vi "Accelerator Read RF Bin quick record 2020 all exec without indicator and warmup.vi"(9 "Sessions Parameters":T2 {"graph_optimization_level" items=["ORT_DISABLE_ALL"=0, "ORT_ENABLE_ALL"=1, "ORT_ENABLE_BASIC"=2, "ORT_ENABLE_EXTENDED"=99]}, 10 "Execution Device":T1=enum."TensorRT", 11 "file path":path=path "C:/Users/COCO/Desktop/TEMP.BIN") -> (3 "exec time":dbl)   [LabVIEW 2020]
uses:
  Source/_Controls/acc_execution_provider_enum.ctl
  Source/Layer/Node/_Controls/acc_onnx_dtype_enum.ctl
  Source/Model/Controls/acc_input_parameters.ctl
  Source/ONNX/_Controls/acc_CUDA_ep_params_simplified.ctl
  Source/ONNX/_Controls/acc_tensorRT_ep_params_simplified.ctl
  Source/Model/_Methods/add_to_graph/Initializer/acc_float_scalar_initializer.vi
  Source/Model/_Methods/add_to_graph/Numeric/acc_div_adaptive.vi
  Source/Model/_Methods/add_to_graph/Complex/Transforms/acc_FFT_optimized.vi
  Source/Model/_Methods/add_to_graph/Initializer/acc_complexfloat_scalar_initializer.vi
  Source/Model/_Methods/add_to_graph/Numeric/acc_mul_adaptive.vi
  Source/Model/_Methods/add_to_graph/Numeric/acc_add_adaptive.vi
  Source/SubVIs/acc_open_netron_from_labview_model.vi
  Source/Model/_Methods/acc_create_onnx_model_then_init_cuda_inference_session.vi
  Source/Model/_Methods/acc_create_onnx_model_then_init_inference_session.vi
  Source/Model/_Methods/acc_create_onnx_model_then_init_tensorRT_inference_session.vi
  Source/ONNX/Inference/_Methods/Simplified/acc_embedded_run_preallocated_mono_input_and_outputs_gpu_by_idx.vi
  Source/ONNX/Inference/_Methods/Exec_GPU/acc_embedded_copy_ptr_data_to_labview_data.vi
  Source/ONNX/Inference/_Methods/Simplified/acc_embedded_run_mono_output_1d_float.vi
  Source/ONNX/Inference/acc_Inference.lvclass
  Source/Model/acc_Model.lvclass
panel:
  out "error out":errorcluster
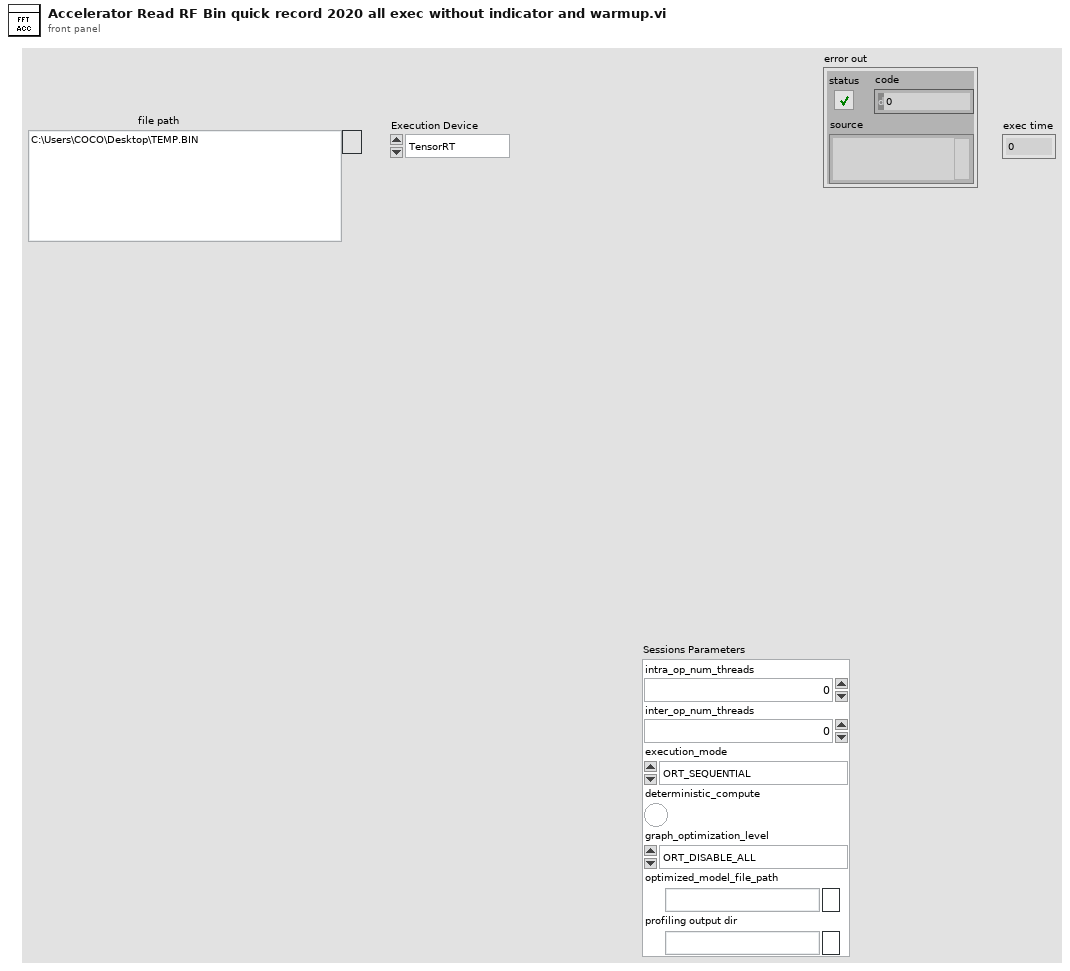
[diagram p1: front panel]
types:
  T1 = typedef "acc_execution_provider_enum.ctl" = enum16{"CPU", "CUDA", "TensorRT"}
  T2 = cluster{"intra_op_num_threads":i32, "inter_op_num_threads":i32, "execution_mode":enum16{"ORT_SEQUENTIAL", "ORT_PARALLEL"}, "deterministic_compute":bool, "graph_optimization_level":u16, "optimized_model_file_path":path, "profiling output dir":path}
  T3 = typedef "acc_input_parameters.ctl" = cluster{"Rank":enum16{"Scalar", "1D", "2D", "3D", "4D", "5D", "6D"}, "dtype":T4, "complex?":bool, "expert?":bool}
  T4 = typedef "acc_onnx_dtype_enum.ctl" = enum16{"UNDEFINED", "FLOAT", "UINT8", "INT8", "UINT16", "INT16", "INT32", "INT64", "STRING", "BOOL", "FLOAT16", "DOUBLE", "UINT32", "UINT64", "COMPLEX64", "COMPLEX128", "BFLOAT16", "FLOAT8E4M3FN", "FLOAT8E4M3FNUZ", "FLOAT8E5M2", "FLOAT8E5M2FNUZ", "UINT4", "INT4"}
  T5 = cluster{"inputs_ptr":u64, "inputs_shapes":i64[], "inputs_ranks":i64, "inputs_types":T4}
  T6 = cluster{"outputs_ptr":u64, "outputs_shapes":i64[], "outputs_ranks":i64, "outputs_types":T4}
  T7 = enum16{"open", "replace", "create", "open or create", "replace or create", "replace or create with confirmation"}
  T8 = typedef "acc_CUDA_ep_params_simplified.ctl" = cluster{"Device & Stream":cluster{"Device Index":i32, "Use Custom Compute Stream?":bool, "Custom Compute Stream (Pointer)":u64, "Copy Using Default Stream?":bool}, "Memory Management":cluster{"GPU Memory Limit (Bytes)":u64, "Arena Extension Strategy":enum16{"kNextPowerOfTwo", "kSameAsRequested"}, "Default Memory Arena Config":u64}, "CuDNN & Kernel Optimization":cluster{"cuDNN Convolution Algorithm Search":enum16{"OrtCudnnConvAlgoSearchExhaustive", "OrtCudnnConvAlgoSearchHeuristic", "OrtCudnnConvAlgoSearchDefault"}, "Use Max Workspace for cuDNN?":bool, "Pad Conv1D Inputs to NC1D?":bool, "Fuse Convolution + Bias?":bool, "Scaled Dot-Product Attention Kernel Option":bool, "Enable Strict SkipLayerNorm Mode?":bool}, "Execution & Precision Controls":cluster{"Enable CUDA Graph Execution?":bool, "Use EP-Level Unified Stream?":bool, "Prefer NHWC Tensor Layout?":bool, "Use TensorFloat-32 (TF32)?":bool}, "Tunable Operator System":cluster{"Enable Tunable Operators?":bool, "Enable Tuning Mode for Tunable Operators?":bool, "Max Tuning Duration (ms)":i32}}
  T9 = typedef "acc_tensorRT_ep_params_simplified.ctl" = cluster{"Device And Stream":cluster{"Device Index":i32, "Use Custom Compute Stream?":bool, "Custom Compute Stream (Pointer)":u64}, "Parser & Subgraph Options":cluster{"Max Partition Attemps":i32, "Minimum Subgraph Size":i32}, "Memory & Workspace Management":cluster{"Max Workspace Memory (Bytes)":u64, "Share Memory Between Subgraphs":bool, "Auxiliary Stream Count":i32}, "Precision & Numeric Modes":cluster{"Enable FP16":bool, "Enable BF16":bool, "Enable INT8":bool, "INT8 Calibration Table Name":path, "Use Native INT8 Calibration?":bool}, "Engine Build, Cache & Paths":cluster{"Enable Engine Caching?":bool, "Engine Cache Directory":path, "Enable Engine Decryption?":bool, "Decryption Library Path":path, "Build Engines Sequentially?":bool, "Enable Timing Cache?":bool, "Timing Cache Directory":path, "Force Timing Cache Use?":bool, "Enable Detailed Logs?":bool, "Use Build Heuristics?":bool, "Enable Weight Sparsity?":bool, "Engine Optimization Level (0–5)":i32}, "Paths & Plugins":cluster{"Extra Plugin Libraries":path[], "Tactic Source Rules":string, "Enabled Preview Features":enum16{"None", "ALIASED_PLUGIN_IO_10_03"}}, "Profile Shapes":cluster{"Minimum Input Shapes":string, "Maximum Input Shapes":string, "Optimal Input Shapes":string}, "Advanced & DLA / CUDA Graph":cluster{"Enable DLA Acceleration?":bool, "DLA Core Index":i32, "Dump TensorRT Subgraphs?":bool, "Force LayerNorm in FP32?":bool, "Enable CUDA Graph Execution?":bool}}
  T10 = enum16{"big-endian, network order", "native, host order", "little-endian"}
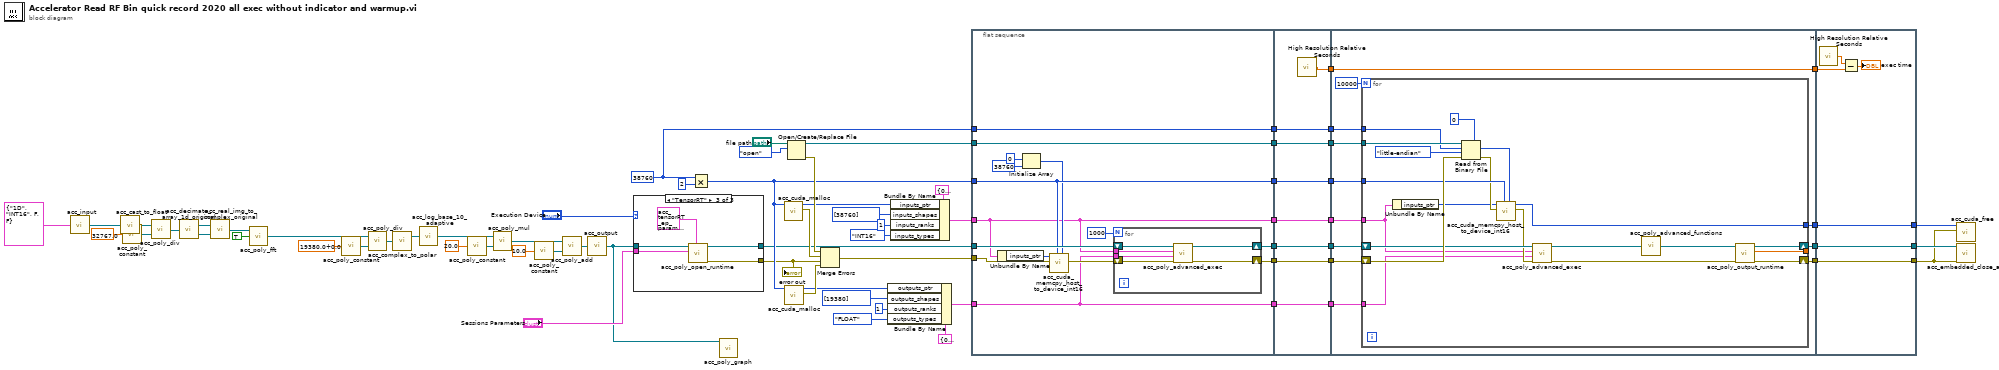
[diagram p0: block diagram]
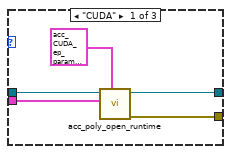
[diagram p2: hidden frame]
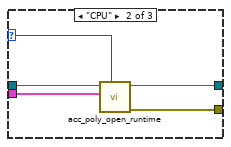
[diagram p3: hidden frame]
diagram:
  w64 = 38760 ("count (1)")
  n1 = call "acc_input.vi"("Parameters"=T3 {"Rank"=enum."1D", "dtype"=enum."INT16", "complex?"=FALSE, "expert?"=FALSE}) -> ("ONNXModel out"=w34:refnum<class "acc_Model.lvclass">)  [unwired: 8 in]
  n2 = call "acc_cast_to_float.vi"("x"=w34) -> ("sgl(x)"=w18:refnum<class "acc_Model.lvclass">)
  n3 = call-poly "acc_poly_constant.vi"("scalar"=sgl 32767.0 ("Numeric")) -> ("Float Scalar"=w16:refnum<class "acc_Model.lvclass">)  [unwired: 3 in]
  n4 = call-poly "acc_poly_div.vi"("y"=w16, "x"=w18) -> ("x/y"=w19:refnum<class "acc_Model.lvclass">)
  n5 = call "acc_decimate_array_1d_original.vi"("array"=w19) -> ("elements 0, n, 2n"=w21:refnum<class "acc_Model.lvclass">, "elements 1, n+1, 2n+1"=w20:refnum<class "acc_Model.lvclass">)
  n6 = call "acc_real_img_to_complex_original.vi"("y"=w20, "x"=w21) -> ("x + iy"=w33:refnum<class "acc_Model.lvclass">)
  n7 = call-poly "acc_poly_fft.vi"("shift?"=TRUE, "X"=w33) -> ("FFT {X}"=w32:refnum<class "acc_Model.lvclass">)  [unwired: 1 in]
  n8 = call-poly "acc_poly_constant.vi"("scalar"=csg 19380.0+0.0i ("Numeric")) -> ("Complex Float Scalar"=w13:refnum<class "acc_Model.lvclass">)  [unwired: 3 in]
  n9 = call-poly "acc_poly_div.vi"("y"=w13, "x"=w32) -> ("x/y"=w26:refnum<class "acc_Model.lvclass">)
  n10 = call "acc_complex_to_polar.vi"("r * e^(i*theta)"=w26) -> ("r"=w22:refnum<class "acc_Model.lvclass">)  [unwired: 1 out]
  n11 = call "acc_log_base_10_adaptive.vi"("x"=w22) -> ("log(x)"=w31:refnum<class "acc_Model.lvclass">)
  n12 = call-poly "acc_poly_constant.vi"("scalar"=sgl 20.0 ("Numeric")) -> ("Float Scalar"=w24:refnum<class "acc_Model.lvclass">)  [unwired: 3 in]
  n13 = call-poly "acc_poly_mul.vi"("y"=w24, "x"=w31) -> ("x*y"=w29:refnum<class "acc_Model.lvclass">)
  n14 = call-poly "acc_poly_constant.vi"("scalar"=sgl 10.0 ("Numeric")) -> ("Float Scalar"=w23:refnum<class "acc_Model.lvclass">)  [unwired: 3 in]
  n15 = call-poly "acc_poly_add.vi"("y"=w23, "x"=w29) -> ("x+y"=w25:refnum<class "acc_Model.lvclass">)
  n16 = call "acc_output.vi"("ONNXModel in"=w25) -> ("ONNXModel out"=w1:refnum<class "acc_Model.lvclass">)  [unwired: 8 in]
  n17 = case shown="\"TensorRT\"" "Execution Device" {
    selector: "Execution Device" -> [_ w77 _]
    tunnel: [w76 w81 w86] -> w5
    tunnel: [w75 w80 w85] -> w4
    tunnel: "Sessions Parameters" -> [w74 w79 w84]
    tunnel: w1 -> [w73 w78 w83]
    frame "CUDA" {
      n18 = call-poly "acc_poly_open_runtime.vi"("CUDA Parameters"=T8 {"Device & Stream"={"Device Index"=0, "Use Custom Compute Stream?"=FALSE, "Custom Compute Stream (Pointer)"=0, "Copy Using Default Stream?"=TRUE}, "Memory Management"={"GPU Memory Limit (Bytes)"=18446744073709551615, "Arena Extension Strategy"=enum."kSameAsRequested", "Default Memory Arena Config"=0}, "CuDNN & Kernel Optimization"={"cuDNN Convolution Algorithm Search"=enum."OrtCudnnConvAlgoSearchHeuristic", "Use Max Workspace for cuDNN?"=FALSE, "Pad Conv1D Inputs to NC1D?"=FALSE, "Fuse Convolution + Bias?"=FALSE, "Scaled Dot-Product Attention Kernel Option"=FALSE, "Enable Strict SkipLayerNorm Mode?"=FALSE}, "Execution & Precision Controls"={"Enable CUDA Graph Execution?"=TRUE, "Use EP-Level Unified Stream?"=FALSE, "Prefer NHWC Tensor Layout?"=FALSE, "Use TensorFloat-32 (TF32)?"=TRUE}, "Tunable Operator System"={"Enable Tunable Operators?"=FALSE, "Enable Tuning Mode for Tunable Operators?"=FALSE, "Max Tuning Duration (ms)"=0}}, "Sessions Parameters"=w74, "Model in"=w73) -> ("error out"=w75:errorcluster, "Inference out"=w76:refnum<class "acc_Inference.lvclass">)  [unwired: 7 in]
    }
    frame "CPU" {
      n19 = call-poly "acc_poly_open_runtime.vi"("Execution Device"=w77, "Sessions Parameters"=w79, "Model in"=w78) -> ("error out"=w80:errorcluster, "Inference out"=w81:refnum<class "acc_Inference.lvclass">)  [unwired: 7 in]
    }
    frame "TensorRT" {
      n20 = call-poly "acc_poly_open_runtime.vi"("TRT Parameters"=T9 {"Device And Stream"={"Device Index"=0, "Use Custom Compute Stream?"=FALSE, "Custom Compute Stream (Pointer)"=0}, "Parser & Subgraph Options"={"Max Partition Attemps"=1000, "Minimum Subgraph Size"=1}, "Memory & Workspace Management"={"Max Workspace Memory (Bytes)"=0, "Share Memory Between Subgraphs"=FALSE, "Auxiliary Stream Count"=-1}, "Precision & Numeric Modes"={"Enable FP16"=FALSE, "Enable BF16"=FALSE, "Enable INT8"=FALSE, "INT8 Calibration Table Name"=path "", "Use Native INT8 Calibration?"=FALSE}, "Engine Build, Cache & Paths"={"Enable Engine Caching?"=FALSE, "Engine Cache Directory"=path "", "Enable Engine Decryption?"=FALSE, "Decryption Library Path"=path "", "Build Engines Sequentially?"=FALSE, "Enable Timing Cache?"=FALSE, "Timing Cache Directory"=path "", "Force Timing Cache Use?"=FALSE, "Enable Detailed Logs?"=FALSE, "Use Build Heuristics?"=FALSE, "Enable Weight Sparsity?"=FALSE, "Engine Optimization Level (0–5)"=3}, "Paths & Plugins"={"Extra Plugin Libraries"=[], "Tactic Source Rules"="", "Enabled Preview Features"=enum."None"}, "Profile Shapes"={"Minimum Input Shapes"="", "Maximum Input Shapes"="", "Optimal Input Shapes"=""}, "Advanced & DLA / CUDA Graph"={"Enable DLA Acceleration?"=FALSE, "DLA Core Index"=0, "Dump TensorRT Subgraphs?"=FALSE, "Force LayerNorm in FP32?"=FALSE, "Enable CUDA Graph Execution?"=FALSE}}, "Sessions Parameters"=w84, "Model in"=w83) -> ("error out"=w85:errorcluster, "Inference out"=w86:refnum<class "acc_Inference.lvclass">)  [unwired: 7 in]
    }
  }
  "error out" <- w4
  n21 = Multiply(x=w64, y=2) -> (x*y=w51:i32)
  n22 = call-poly "acc_poly_graph.vi"("Model"=w1) -> ()  [unwired: 13 in, 2 out]
  n23 = call "acc_cuda_malloc.vi"("size (bytes)"=w51) -> ("error out"=w50:errorcluster, "devPtr"=w40:u64)  [unwired: 9 in]
  n24 = call "acc_cuda_malloc.vi"("size (bytes)"=w51) -> ("error out"=w49:errorcluster, "devPtr"=w47:u64)  [unwired: 9 in]
  n25 = Open/Create/Replace File(file path (use dialog)="file path", operation (0:open)=T7."open") -> (refnum out=w68:refnum<file>, error out=w66:errorcluster)  [unwired: 4 in, 1 out]
  n26 = Merge Errors(w66, w50, w4, w49) -> (w67:errorcluster)
  n27 = Bundle By Name(cluster=T6 {"outputs_ptr"=0, "outputs_shapes"=[], "outputs_ranks"=0, "outputs_types"=enum."UNDEFINED"} ("Outputs Info"), "outputs_ptr"=w47, "outputs_shapes"=i64[] [19380] ("inputs_shapes"), "outputs_ranks"=i64 1, "outputs_types"=acc_onnx_dtype_enum."FLOAT") -> (w42:T6)
  n28 = Bundle By Name(cluster=T5 {"inputs_ptr"=0, "inputs_shapes"=[], "inputs_ranks"=0, "inputs_types"=enum."UNDEFINED"} ("Inputs Info"), "inputs_ptr"=w40, "inputs_shapes"=i64[] [38760], "inputs_ranks"=i64 1, "inputs_types"=acc_onnx_dtype_enum."INT16") -> (w35:T5)
  n29 = flat-sequence {
    tunnel: w35 -> [w88]
    tunnel: w42 -> [w87]
    tunnel: w5 -> [w99]
    tunnel: w64 -> [w100]
    tunnel: w51 -> [w94]
    tunnel: w67 -> [w96]
    tunnel: w68 -> [w101]
    tunnel: [w101] -> w12
    tunnel: [w98] -> w11
    tunnel: [w94] -> w10
    tunnel: [w100] -> w9
    tunnel: [w87] -> w8
    tunnel: [w88] -> w7
    tunnel: [w97] -> w6
    tunnel: [w115] -> w61
    tunnel: [w114] -> w60
    tunnel: [w113] -> w59
    tunnel: [w112] -> w58
    tunnel: [w111] -> w57
    tunnel: [w110] -> w53
    tunnel: [w109] -> w43
    tunnel: [w108] -> w36
    tunnel: w12 -> [w115]
    tunnel: w11 -> [w114]
    tunnel: w10 -> [w113]
    tunnel: w9 -> [w112]
    tunnel: w8 -> [w109]
    tunnel: w7 -> [w108]
    tunnel: w6 -> [w111]
    tunnel: w61 -> [w125]
    tunnel: w60 -> [w124]
    tunnel: w59 -> [w123]
    tunnel: w58 -> [w122]
    tunnel: w57 -> [w119]
    tunnel: [w127] -> w56
    tunnel: [w121] -> w55
    tunnel: [w120] -> w54
    tunnel: w53 -> [w118]
    tunnel: [w118] -> w52
    tunnel: w43 -> [w117]
    tunnel: w36 -> [w116]
    tunnel: [w151] -> w62
    tunnel: [w152] -> w63
    tunnel: [w153] -> w69
    tunnel: w56 -> [w153]
    tunnel: w55 -> [w152]
    tunnel: w54 -> [w151]
    tunnel: w52 -> [w149]
    frame #0 {
      n30 = Unbundle By Name(w88) -> ("inputs_ptr"=w89:u64)
      n31 = Initialize Array(i16 0 ("element"), i64 38760 ("Numeric")) -> (w90:i16[])
      n32 = call "acc_cuda_memcpy_host_to_device_int16.vi"("data"=w90, "size"=w94, "error in"=w96, "devPtr"=w89) -> ("error out"=w95:errorcluster)  [unwired: 6 in, 1 out]
      n33 = for {
        N: 1000 -> [_]
        shift-right: [w105] -> w98
        shift-left: w95 -> [w107]
        shift-right: [w104] -> w97
        shift-left: w99 -> [w106]
        tunnel: w88 -> [w103]
        tunnel: w87 -> [w102]
        n34 = call-poly "acc_poly_advanced_exec.vi"("error in"=w107, "Outputs Info"=w102, "Inputs Info"=w103, "Inference in"=w106) -> ("error out"=w105:errorcluster, "Inference out"=w104:refnum<class "acc_Inference.lvclass">)  [unwired: 6 in]
      }
    }
    frame #1 {
      n35 = call <vilib>:"High Resolution Relative Seconds.vi"() -> ("relative seconds"=w110:dbl)
    }
    frame #2 {
      n36 = for {
        N: 10000 -> [_]
        shift-right: [w139] -> w127
        shift-left: w119 -> [w143]
        shift-right: [w140] -> w121
        shift-left: w124 -> [w147]
        tunnel: w125 -> [w146]
        tunnel: w123 -> [w145]
        tunnel: w122 -> [w144]
        tunnel: [w138] -> w120
        tunnel: w117 -> [w131]
        tunnel: w116 -> [w129]
        tunnel: [w128] -> _
        n37 = Unbundle By Name(w129) -> ("inputs_ptr"=w130:u64)
        n38 = Read from Binary File(5:i16 0 ("Numeric"), 8:w147, 9:T10."little-endian" ("byte order (0:big-endian, network order)"), 10:w144, 11:w146) -> (0:w137:errorcluster, 2:w134:i16[])  [unwired: 1 in, 2 out]
        n39 = call "acc_cuda_memcpy_host_to_device_int16.vi"("data"=w134, "size"=w145, "error in"=w137, "devPtr"=w130) -> ("error out"=w132:errorcluster, "dup devPtr"=w138:u64)  [unwired: 6 in]
        n40 = call-poly "acc_poly_advanced_exec.vi"("error in"=w132, "Outputs Info"=w131, "Inputs Info"=w129, "Inference in"=w143) -> ("error out"=w142:errorcluster, "Inference out"=w141:refnum<class "acc_Inference.lvclass">)  [unwired: 6 in]
        n41 = call-poly "acc_poly_advanced_functions.vi"("Inference in"=w141) -> ("Inference out"=w133:refnum<class "acc_Inference.lvclass">)
        n42 = call-poly "acc_poly_output_runtime.vi"("error in"=w142, "Inference in"=w133) -> ("error out"=w140:errorcluster, "1D Output Data"=w128:sgl[], "Inference out"=w139:refnum<class "acc_Inference.lvclass">)  [unwired: 7 in]
      }
    }
    frame #3 {
      n43 = call <vilib>:"High Resolution Relative Seconds.vi"() -> ("relative seconds"=w150:dbl)
      n44 = Subtract(x=w150, y=w149) -> (x-y=→"exec time":dbl)
    }
  }
  n45 = call "acc_cuda_free.vi"("error in"=w63, "devPtr"=w62) -> ()  [unwired: 9 in, 1 out]
  n46 = call-dynamic "acc_embedded_close_all.vi"("error in"=w63, "Inference in"=w69) -> ()  [unwired: 8 in, 2 out]
